vi "create SimpleSavings.vi"(4 "Interest Rate Interval (s)":u32, 6 "Interest Rate":dbl, 7 "Account Number":string, 8 "error in (no error)":errorcluster, 10 "Initial Balance":dbl, 11 "SimpleSavings in":refnum<class "SimpleSavings.lvclass">) -> (0 "error out":errorcluster, 3 "SimpleSavings out":refnum<class "SimpleSavings.lvclass">)   [LabVIEW 2020, in "SimpleSavings.lvclass"]
uses:
  SimpleSavings.lvclass
  C:/projects/budget_LabVIEW/Main Codeline/Software/Code/shared/AAccount/AAccount.lvclass
  C:/projects/budget_LabVIEW/Main Codeline/Software/Code/shared/AInterestAccount/AInterestAccount.lvclass
  SimpleSavings.lvclass/SimpleSavings.ctl
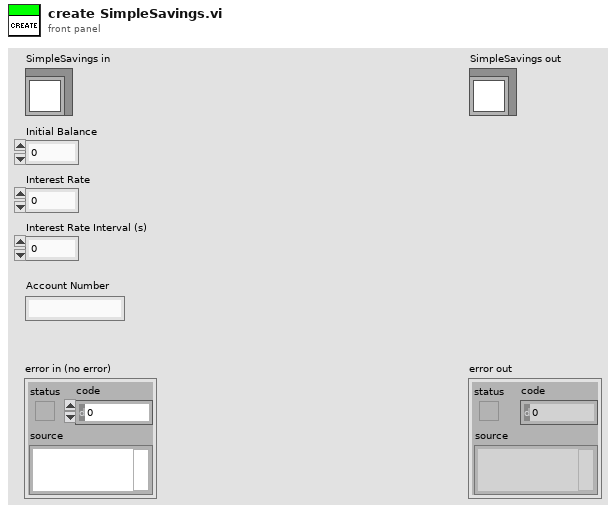
[diagram p1: front panel]
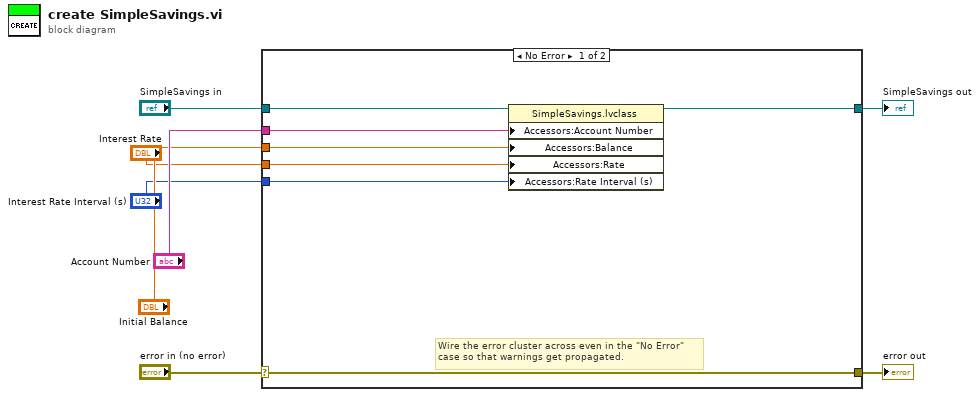
[diagram p0: block diagram]
diagram:
  n1 = case shown="No Error" "error in (no error)" {
    selector: "error in (no error)" -> [w14 w17]
    tunnel: [w14 w17] -> w7
    tunnel: [w13 w16] -> w5
    tunnel: "SimpleSavings in" -> [w15 w16]
    tunnel: "Account Number" -> [w12 _]
    tunnel: "Initial Balance" -> [w11 _]
    tunnel: "Interest Rate" -> [w10 _]
    tunnel: "Interest Rate Interval (s)" -> [w9 _]
    frame No Error {
      # "Wire the error cluster across even in the \"No Error\"\ncase so that warnings get propagated."
      n2 = property class="SimpleSavings.lvclass"(reference=w15, "Accessors:Account Number"=w12, "Accessors:Balance"=w11, "Accessors:Rate"=w10, "Accessors:Rate Interval (s)"=w9) -> (reference out=w13:refnum<class "SimpleSavings.lvclass">)  [unwired: 1 in, 1 out]
    }
    frame Error {
    }
  }
  "error out" <- w7
  "SimpleSavings out" <- w5
